vi "FRCts20_Backend_ObtainReturn.vi"(6 "Timeout (ms, 10000)":i32=10000, 8 "error in (no error)":errorcluster, 9 "Key":string) -> (0 "error out":errorcluster, 3 "Message Value":string)   [LabVIEW 2013, in "FRCts20_Backend_Engine.lvlib"]
doc: "Dequeue provides a generic function handle for retrieving data from the returns queue. The function systematically checks for <b>Key ID</b> match, and returns <b>raw message byte string</b>. The caller is responsible for the appropriate un-flatten step."
uses:
  FRCts20_Backend_Engine.lvlib
  FRCts20_Backend_DequeueDataOperations.ctl
  FRCts20_Backend_FGVOperation.ctl
panel:
  # "Dequeue provides a generic function handle for \nretrieving data from the returns queue. Systematically\nchecks for Key ID match, and returns raw message \nstring. The caller is responsible for the appropriate un-\nflatten step."
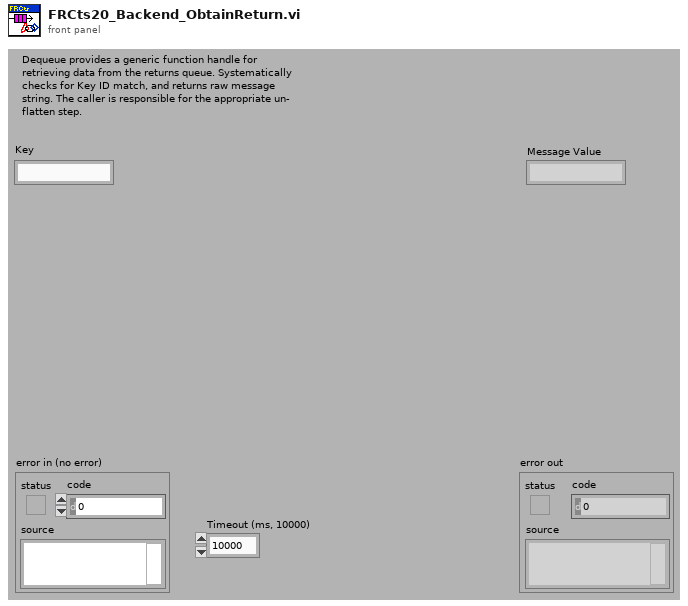
[diagram p1: front panel]
types:
  T1 = typedef "FRCts20_Backend_Engine.lvlib/FRCts20_Backend_DequeueDataOperations.ctl" = enum16{"Initialize", "DequeueDataReturn", "GetQueues"}
  T2 = typedef "FRCts20_Backend_Engine.lvlib/FRCts20_Backend_FGVOperation.ctl" = enum16{"Initialize", "EnqueueMessage", "EnqueueDataReturn", "FlushMessage", "FlushDataReturn"}
  T3 = typedef "FRCts20_Backend_Engine.lvlib/FRCts20_Backend_EngineRefnums.ctl" = cluster{"Message Queue Methods":T4, "Message Queue Returns":T4, "Data Store Path":path, "Database Refnum":T5, "INI":refnum<class "FRCts20_Backend_INI Controller.lvclass">}
  T4 = typedef "AMC.lvlib/Message Queue.ctl" = refnum<queue>
  T5 = typedef "NI_Database_API.lvlib/Conn ObjectReference.ctl" = refnum<k1>
  T6 = typedef "AMC.lvlib/Message.ctl" = cluster{"Name":string, "Value":string, "Attributes":T7, "Receiver Host":string, "Receiver Process":string, "Source Host":string, "Source Process":string, "Priority Message":bool, "Acknowledge Message":bool}
  T7 = typedef "Tools_KeyedArray.lvlib/KeyedArray.ctl" = cluster{"keys":string[], "values":string[]}
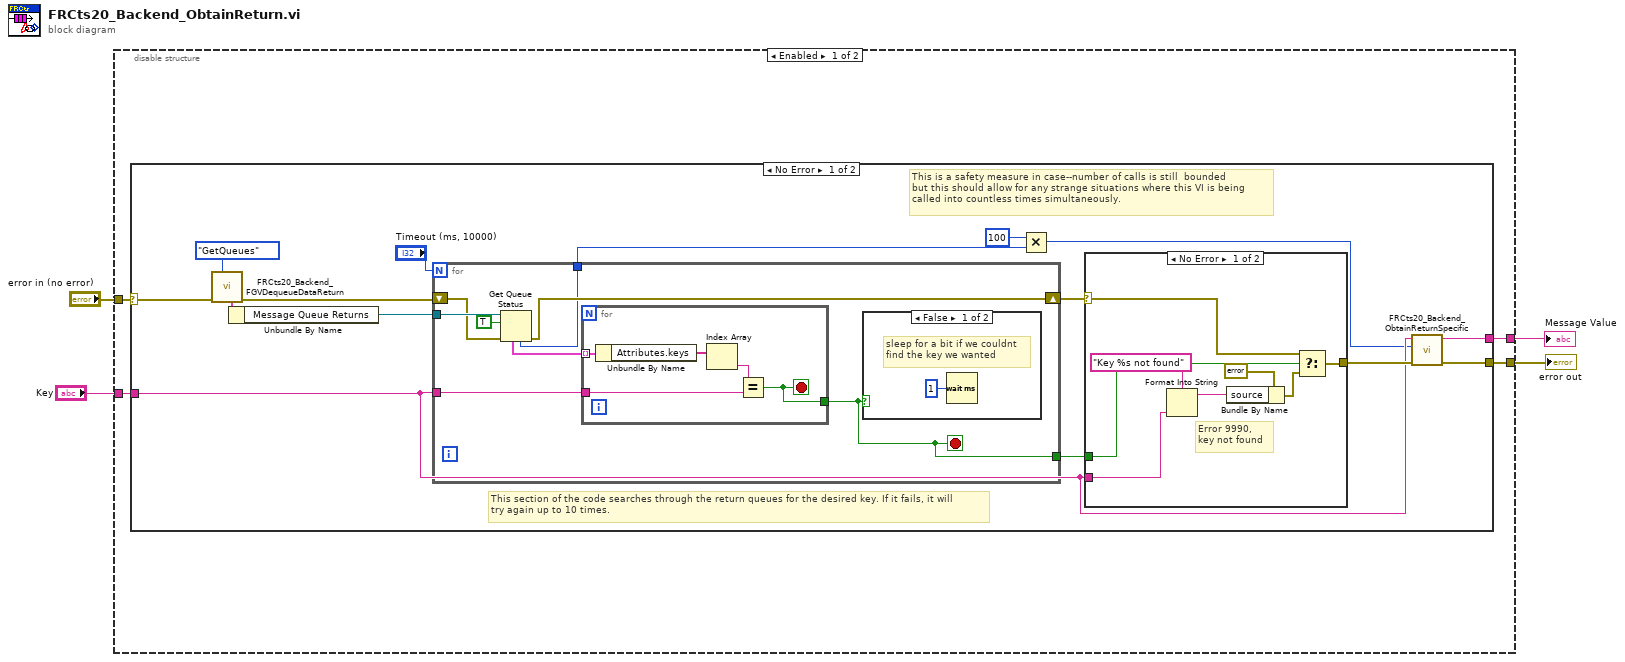
[diagram p0: block diagram]
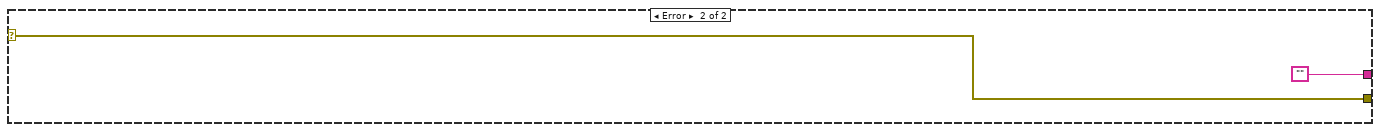
[diagram p4: hidden frame]
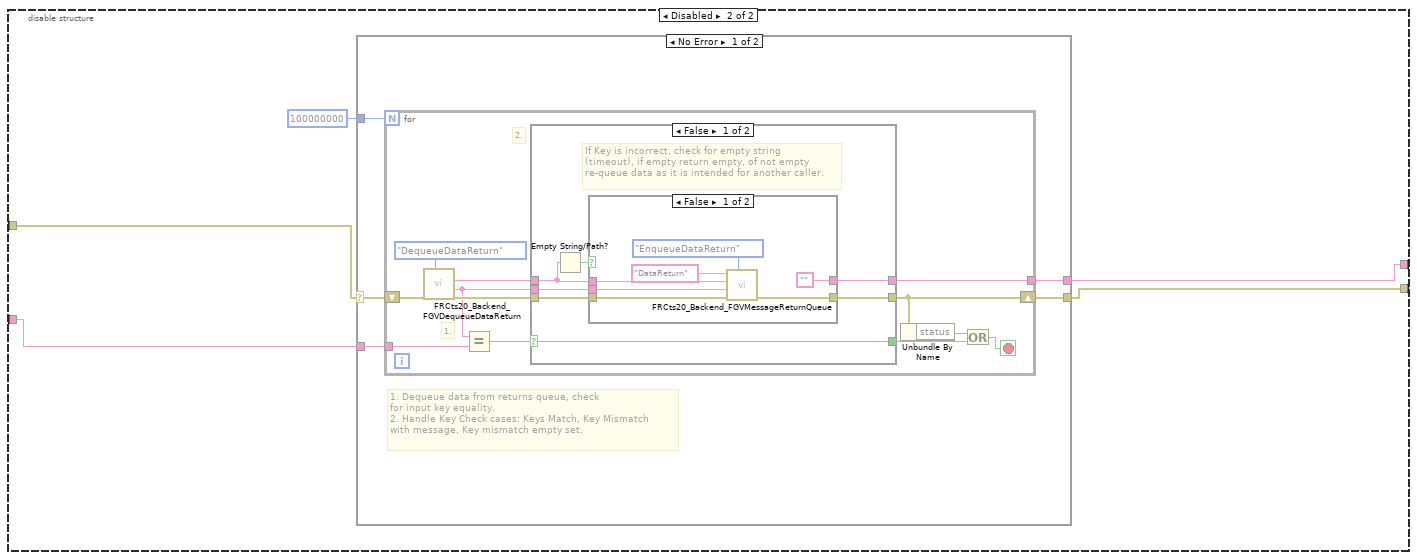
[diagram p5: hidden frame]
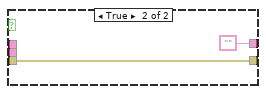
[diagram p6: hidden frame]
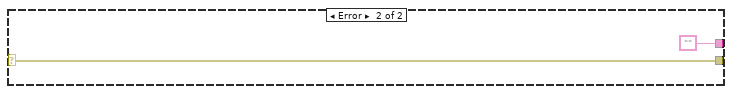
[diagram p8: hidden frame]
diagram:
  n1 = disable-structure shown="Enabled" {
    disable-tunnel: "error in (no error)" -> [w8 w52]
    disable-tunnel: [w7 w49] -> w3
    disable-tunnel: [w6 w50] -> w2
    disable-tunnel: "Key" -> [w5 w53]
    frame Enabled {
      n2 = case shown="No Error" w8 {
        selector: w8 -> [w19 w47]
        tunnel: [w14 ""] -> w6
        tunnel: [w13 w47] -> w7
        tunnel: w5 -> [w11 _]
        frame No Error {
          # "This section of the code searches through the return queues for the desired key. If it fails, it will\ntry again up to 10 times."
          # "This is a safety measure in case--number of calls is still  bounded\nbut this should allow for any strange situations where this VI is being\ncalled into countless times simultaneously."
          n3 = call "FRCts20_Backend_FGVDequeueDataReturn.vi"("Operation"=FRCts20_Backend_DequeueDataOperations."GetQueues", "error in (no error)"=w19) -> ("error out"=w18:errorcluster, "Engine_Refnums Out"=w22:T3)  [unwired: 5 in, 3 out]
          n4 = Unbundle By Name(w22) -> ("Message Queue Returns"=w21:T4)
          n5 = for {
            N: "Timeout (ms, 10000)" -> [_]
            tunnel: w21 -> [w40]
            tunnel: w11 -> [w37]
            tunnel: [w36] -> w16
            shift-right: [w34] -> w17
            shift-left: w18 -> [w35]
            tunnel: [w33] -> w12
            stop <- w36 stop-if-true
            n6 = Get Queue Status(queue=w40, return elements? (F)=TRUE, error in (no error)=w35) -> (error out=w34:errorcluster, # elements in queue=w33:i32, elements=w38:T6[])  [unwired: 5 out]
            n7 = for {
              tunnel: w38 -> [w46] mode=indexing
              tunnel: w37 -> [w43]
              tunnel: [w42] -> w36
              stop <- w42 stop-if-true
              n8 = Unbundle By Name(w46) -> ("Attributes.keys"=w45:string[])
              n9 = Index Array(array=w45) -> (element=w44:string)  [unwired: 1 in]
              n10 = Equal?(x=w44, y=w43) -> (x = y?=w42:bool)
            }
            n11 = case shown="False" w36 {
              frame False {
                # "sleep for a bit if we couldnt\nfind the key we wanted"
                n12 = Wait (ms)(milliseconds to wait=u32 1) -> ()  [unwired: 1 out]
              }
              frame True {
                # "Found key value\nin queue, do nothing\njust yet"
              }
            }
          }
          n13 = Multiply(x=100, y=w12) -> (x*y=w10:i32)
          n14 = case shown="No Error" w17 {
            selector: w17 -> [w30 w32]
            tunnel: w16 -> [w31 _]
            tunnel: w11 -> [w27 _]
            tunnel: [w24 w32] -> w15
            frame No Error {
              # "Error 9990,\nkey not found"
              n15 = Format Into String(format string="Key %s not found", w27) -> (resulting string=w25:string)  [unwired: 2 in, 1 out]
              n16 = Bundle By Name(cluster=errorcluster {"status"=TRUE, "code"=9990, "source"=""} ("f"), "source"=w25) -> (w28:errorcluster)
              n17 = Select(t=w30, s=w31, f=w28) -> (s? t:f=w24:errorcluster)
            }
            frame Error {
            }
          }
          n18 = call "FRCts20_Backend_ObtainReturnSpecific.vi"("error in (no error)"=w15, "Elements to search"=w10, "Key in"=w11) -> ("error out"=w13:errorcluster, "Message Value"=w14:string)  [unwired: 7 in]
        }
        frame Error {
        }
      }
    }
    frame Disabled {
      n19 = case shown="No Error" w52 {
        selector: w52 -> [w58 w91]
        tunnel: [w57 w91] -> w49
        tunnel: w53 -> [w56 _]
        tunnel: [w55 ""] -> w50
        tunnel: 100000000 ("Elements to search") -> [w54 _]
        frame No Error {
          # "1. Dequeue data from returns queue, check\nfor input key equality.\n2. Handle Key Check cases: Keys Match, Key Mismatch\nwith message, Key mismatch empty set."
          n20 = for {
            N: w54 -> [_]
            shift-right: [w65] -> w57
            shift-left: w58 -> [w70]
            tunnel: w56 -> [w68]
            tunnel: [w60] -> w55
            stop <- w59 stop-if-true
            # "2."
            # "1."
            n21 = call "FRCts20_Backend_FGVDequeueDataReturn.vi"("Operation"=FRCts20_Backend_DequeueDataOperations."DequeueDataReturn", "error in (no error)"=w70) -> ("error out"=w66:errorcluster, "Key"=w61:string, "Message Value"=w62:string)  [unwired: 5 in, 2 out]
            n22 = Equal?(x=w61, y=w68) -> (x = y?=w67:bool)
            n23 = case shown="False" w67 {
              selector: w67 -> [w72 w88]
              tunnel: w66 -> [w76 w89]
              tunnel: [w75 w89] -> w65
              tunnel: [w72 w88] -> w63
              tunnel: w62 -> [w73 w87]
              tunnel: [w74 w87] -> w60
              tunnel: w61 -> [w71 _]
              frame False {
                # "If Key is incorrect, check for empty string \n(timeout), if empty return empty, of not empty\nre-queue data as it is intended for another caller."
                n24 = Empty String/Path?(string/path=w73) -> (empty?=w77:bool)
                n25 = case shown="False" w77 {
                  tunnel: w76 -> [w84 w86]
                  tunnel: [w83 w86] -> w75
                  tunnel: ["" ""] -> w74
                  tunnel: w73 -> [w81 _]
                  tunnel: w71 -> [w78 _]
                  frame False {
                    n26 = call "FRCts20_Backend_FGVMessageReturnQueue.vi"("Operation"=FRCts20_Backend_FGVOperation."EnqueueDataReturn", "error in (no error)"=w84, "Key"=w78, "Message Value"=w81, "Message Name"="DataReturn") -> ("error out"=w83:errorcluster)  [unwired: 5 in, 1 out]
                  }
                  frame True {
                  }
                }
              }
              frame True {
                # "If Key is correct, return Message Value\nto the caller."
              }
            }
            n27 = Unbundle By Name(w65) -> ("status"=w64:bool)
            n28 = Or(x=w64, y=w63) -> (x .or. y?=w59:bool)
          }
        }
        frame Error {
        }
      }
    }
  }
  "error out" <- w3
  "Message Value" <- w2
